vi "DCA Determine Switch Configuration.vi"(1 "Measurement":T1) -> (0 "SWI Position":T2)   [LabVIEW 2011]
uses:
  drivers/SWI/Sea-Level/TypeDefs/Sea-Level SWI Position.ctl
  TypeDefs/DCA Measurement.ctl
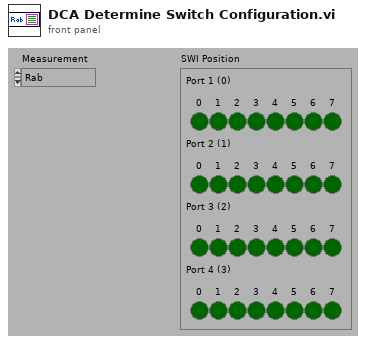
[diagram p1: front panel]
types:
  T1 = typedef "DCA Measurement.ctl" = enum16{"Rab", "Rac", "Rbc"}
  T2 = typedef "Sea-Level SWI Position.ctl" = cluster{"Port 1 (0)":cluster{"0":bool, "1":bool, "2":bool, "3":bool, "4":bool, "5":bool, "6":bool, "7":bool}, "Port 2 (1)":cluster{"0":bool, "1":bool, "2":bool, "3":bool, "4":bool, "5":bool, "6":bool, "7":bool}, "Port 3 (2)":cluster{"0":bool, "1":bool, "2":bool, "3":bool, "4":bool, "5":bool, "6":bool, "7":bool}, "Port 4 (3)":cluster{"0":bool, "1":bool, "2":bool, "3":bool, "4":bool, "5":bool, "6":bool, "7":bool}}
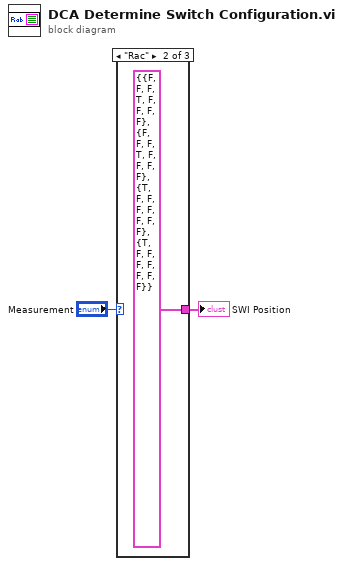
[diagram p0: block diagram]
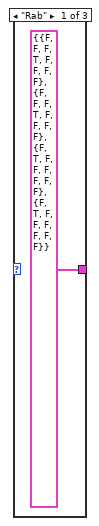
[diagram p2: hidden frame]
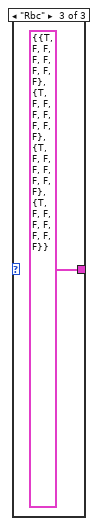
[diagram p3: hidden frame]
diagram:
  n1 = case shown="\"Rac\"" "Measurement" {
    tunnel: [T2 {"Port 1 (0)"={"0"=FALSE, "1"=FALSE, "2"=FALSE, "3"=TRUE, "4"=FALSE, "5"=FALSE, "6"=FALSE, "7"=FALSE}, "Port 2 (1)"={"0"=FALSE, "1"=FALSE, "2"=FALSE, "3"=TRUE, "4"=FALSE, "5"=FALSE, "6"=FALSE, "7"=FALSE}, "Port 3 (2)"={"0"=FALSE, "1"=TRUE, "2"=FALSE, "3"=FALSE, "4"=FALSE, "5"=FALSE, "6"=FALSE, "7"=FALSE}, "Port 4 (3)"={"0"=FALSE, "1"=TRUE, "2"=FALSE, "3"=FALSE, "4"=FALSE, "5"=FALSE, "6"=FALSE, "7"=FALSE}} T2 {"Port 1 (0)"={"0"=FALSE, "1"=FALSE, "2"=FALSE, "3"=TRUE, "4"=FALSE, "5"=FALSE, "6"=FALSE, "7"=FALSE}, "Port 2 (1)"={"0"=FALSE, "1"=FALSE, "2"=FALSE, "3"=TRUE, "4"=FALSE, "5"=FALSE, "6"=FALSE, "7"=FALSE}, "Port 3 (2)"={"0"=TRUE, "1"=FALSE, "2"=FALSE, "3"=FALSE, "4"=FALSE, "5"=FALSE, "6"=FALSE, "7"=FALSE}, "Port 4 (3)"={"0"=TRUE, "1"=FALSE, "2"=FALSE, "3"=FALSE, "4"=FALSE, "5"=FALSE, "6"=FALSE, "7"=FALSE}} T2 {"Port 1 (0)"={"0"=TRUE, "1"=FALSE, "2"=FALSE, "3"=FALSE, "4"=FALSE, "5"=FALSE, "6"=FALSE, "7"=FALSE}, "Port 2 (1)"={"0"=TRUE, "1"=FALSE, "2"=FALSE, "3"=FALSE, "4"=FALSE, "5"=FALSE, "6"=FALSE, "7"=FALSE}, "Port 3 (2)"={"0"=TRUE, "1"=FALSE, "2"=FALSE, "3"=FALSE, "4"=FALSE, "5"=FALSE, "6"=FALSE, "7"=FALSE}, "Port 4 (3)"={"0"=TRUE, "1"=FALSE, "2"=FALSE, "3"=FALSE, "4"=FALSE, "5"=FALSE, "6"=FALSE, "7"=FALSE}}] -> w1
    frame "Rab" {
    }
    frame "Rac" {
    }
    frame "Rbc" {
    }
  }
  "SWI Position" <- w1
